vi "addOne.vi"(8 "error in (no error)":errorcluster, 11 "input":dbl) -> (0 "error out":errorcluster, 3 "value":dbl)   [LabVIEW 2018]
doc: "Addition with one fucntion for the test purpose."
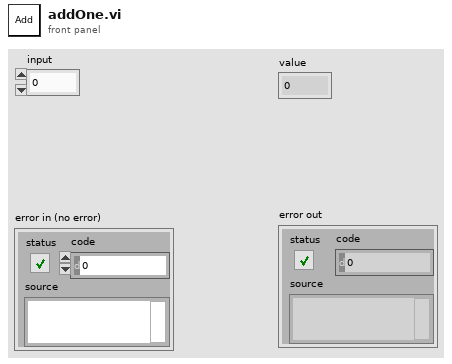
[diagram p1: front panel]
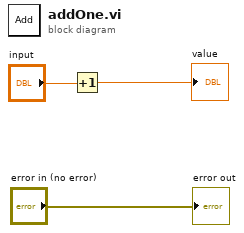
[diagram p0: block diagram]
diagram:
  n1 = Increment(x="input") -> (x+1=→"value":dbl)
  "error out" <- "error in (no error)"
